vi "Search Bookmarks with event names Broadcasts.vi"(8 "error in":errorcluster, 10 "VIs to Search for Bookmarks Paths":path[](array[path]), 11 "Application in":refnum<vi>) -> (0 "error out":errorcluster)   [LabVIEW 2016, in "PantherLAB_Scripting.lvlib"]
uses:
  PantherLAB_Scripting.lvlib
  <vilib>/Utility/traverseref.llb/TRef TravTarget.ctl
  <vilib>/Utility/traverseref.llb/VI Scripting - Traverse.lvlib
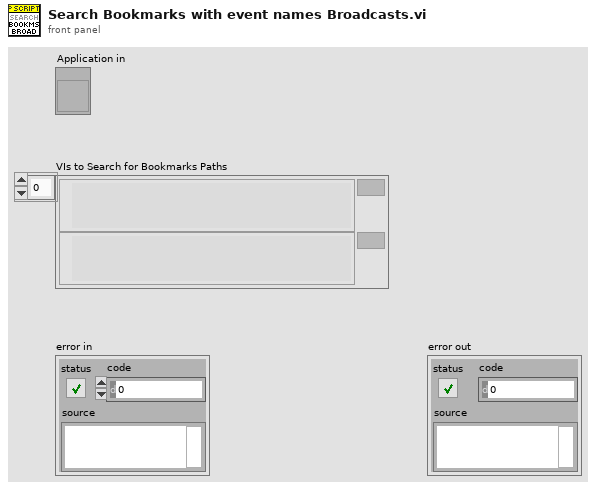
[diagram p1: front panel]
types:
  T1 = typedef "TRef TravTarget.ctl" = enum16{"FP", "BD", "Other"}
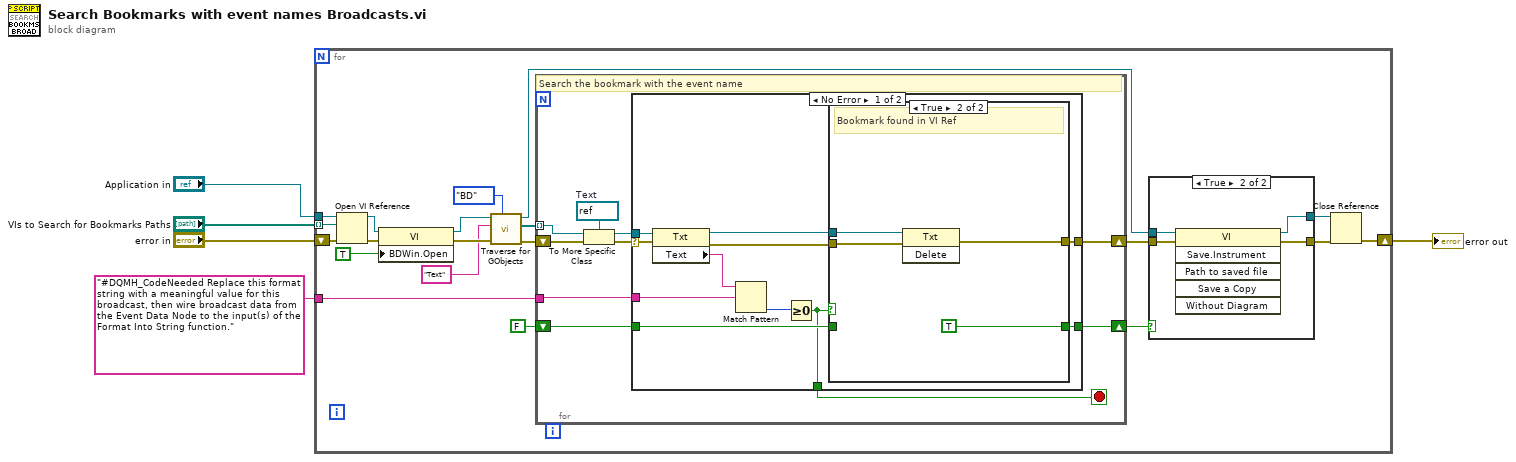
[diagram p0: block diagram]
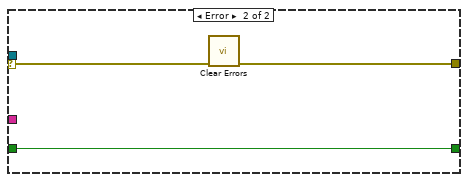
[diagram p3: hidden frame]
diagram:
  n1 = for {
    tunnel: "Application in" -> [w13]
    tunnel: "#DQMH_CodeNeeded Replace this format string with a meaningful value for this broadcast, then wire broadcast data from the Event Data Node to the input(s) of the Format Into String function." -> [w11]
    tunnel: "VIs to Search for Bookmarks Paths" -> [w10] mode=indexing
    shift-right: [w20] -> w5
    shift-left: "error in" -> [w21]
    n2 = Open VI Reference(application reference (local)=w13, vi path=w10, error in (no error)=w21) -> (vi reference=w15:refnum<vi>, error out=w23:errorcluster)  [unwired: 3 in]
    n3 = property class="VI"(reference=w15, error in=w23, "BDWin.Open"=TRUE ("Block Diagram Window:Open")) -> (reference out=w14:refnum<vi>, error out=w22:errorcluster)
    n4 = call <vilib>:"Traverse for GObjects.vi"("Traverse Target"=TRef_TravTarget."BD", "error in (no error)"=w22, "Class Name"="Text", "VI Refnum"=w14) -> ("error out"=w25:errorcluster, "References"=w12:refnum<vi>[], "dup VI Refnum"=w8:refnum<vi>)  [unwired: 4 in, 1 out]
    n5 = for {
      shift-right: [w34] -> w24
      shift-left: w25 -> [w35]
      tunnel: w12 -> [w31] mode=indexing
      tunnel: w11 -> [w27]
      shift-right: [w28] -> w6
      shift-left: FALSE -> [w29]
      stop <- w26 stop-if-true
      w32 = refnum<vi> refnum  # Text
      # "Search the bookmark with the event name"
      n6 = To More Specific Class(target class=w32, reference=w31, error in=w35) -> (specific class reference=w30:refnum<vi>, error out=w33:errorcluster)
      n7 = case shown="No Error" w33 {
        selector: w33 -> [w45 w55]
        tunnel: [w46 w54] -> w34
        tunnel: w30 -> [w43 _]
        tunnel: w29 -> [w40 w53]
        tunnel: [w39 w53] -> w28
        tunnel: w27 -> [w37 _]
        tunnel: [w36 _] -> w26
        frame No Error {
          n8 = property class="Txt"(reference=w43, error in=w45) -> (reference out=w41:refnum<vi>, error out=w44:errorcluster, "Text"=w42:string)
          n9 = Match Pattern(string=w42, regular expression=w37) -> (offset past match=w38:i32)  [unwired: 1 in, 3 out]
          n10 = Greater Or Equal To 0?(x=w38) -> (x >= 0?=w36:bool)
          n11 = case shown="True" w36 {
            tunnel: w44 -> [w48 w49]
            tunnel: w41 -> [_ w50]
            tunnel: [w48 w52] -> w46
            tunnel: w40 -> [w47 _]
            tunnel: [w47 TRUE] -> w39
            frame False {
              # "Text Not Found"
            }
            frame True {
              # "Bookmark found in VI Ref"
              n12 = invoke class="Txt" method="Delete"(reference=w50, error in=w49) -> (error out=w52:errorcluster)  [unwired: 1 in, 2 out]
            }
          }
        }
        frame Error {
          n13 = call <vilib>:"Clear Errors.vi"("error in (no error)"=w55) -> ("error out"=w54:errorcluster)  [unwired: 5 in, 1 out]
        }
      }
    }
    n14 = case shown="True" w6 {
      tunnel: w24 -> [w57 w61]
      tunnel: [w57 w60] -> w19
      tunnel: w8 -> [w56 w59]
      tunnel: [w56 w58] -> w7
      frame False {
      }
      frame True {
        n15 = invoke class="VI" method="Save.Instrument"(reference=w59, error in=w61) -> (reference out=w58:refnum<vi>, error out=w60:errorcluster)  [unwired: 4 in, 4 out]
      }
    }
    n16 = Close Reference(reference=w7, error in (no error)=w19) -> (error out=w20:errorcluster)
  }
  "error out" <- w5
